vi "Write DistanceToDrive.vi"(8 "error in (no error)":errorcluster, 10 "DistanceToDrive":dbl, 11 "DM-DriveForwardDistance in":refnum<class "DM-DriveForwardDistance.lvclass">) -> (0 "error out":errorcluster, 3 "DM-DriveForwardDistance out":refnum<class "DM-DriveForwardDistance.lvclass">)   [LabVIEW 2013, in "DM-DriveForwardDistance.lvclass"]
uses:
  DM-DriveForwardDistance.lvclass
  DM-DriveForwardDistance.lvclass/DM-DriveForwardDistance.ctl
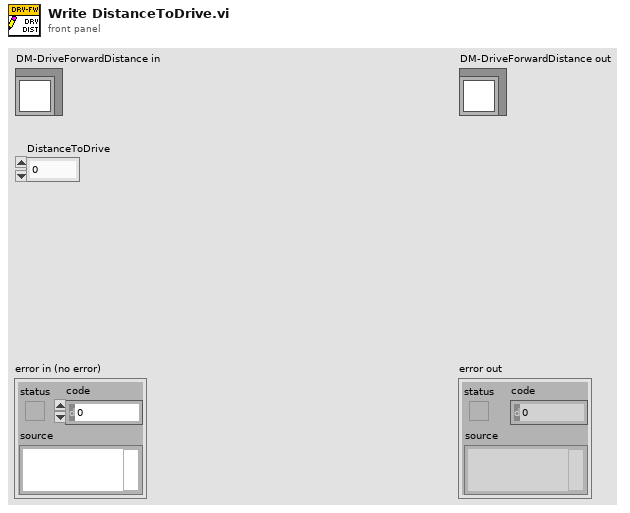
[diagram p1: front panel]
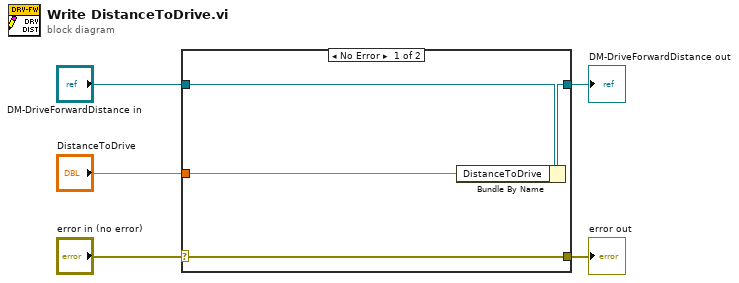
[diagram p0: block diagram]
diagram:
  n1 = case shown="No Error" "error in (no error)" {
    selector: "error in (no error)" -> [w9 w10]
    tunnel: [w9 w10] -> w4
    tunnel: [w7 w11] -> w2
    tunnel: "DM-DriveForwardDistance in" -> [w8 w11]
    tunnel: "DistanceToDrive" -> [w6 _]
    frame No Error {
      n2 = Bundle By Name(cluster=w8, "DistanceToDrive"=w6) -> (w7:refnum<class "DM-DriveForwardDistance.lvclass">)
    }
    frame Error {
    }
  }
  "error out" <- w4
  "DM-DriveForwardDistance out" <- w2
